vi "20211001_02.vi"() -> ()   [LabVIEW 2019]
uses:
  <vilib>/Utility/miscctls.llb/LVBoundsTypeDef.ctl
panel:
  in  "Button Size":T1={"Width"=192, "Height"=192}
  in  "Visible":bool=TRUE
  in  "Colors [4]":cluster{"Color Box":u32, "Color Box 2":u32}[](array[cluster])=[{"Color Box"=16777216, "Color Box 2"=16777216}, {"Color Box"=4424887, "Color Box 2"=4424887}, {"Color Box"=16777216, "Color Box 2"=16777216}, {"Color Box"=4424887, "Color Box 2"=4424887}]
  in  "Boolean":bool
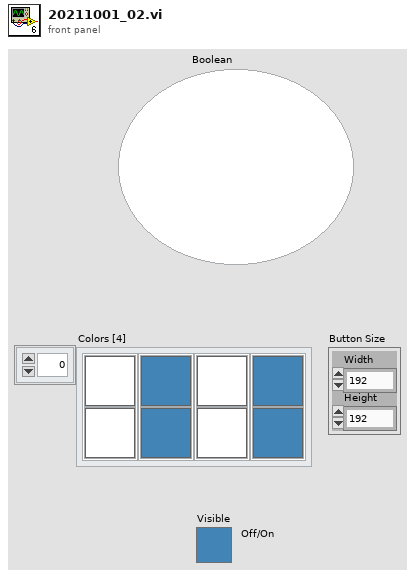
[diagram p1: front panel]
types:
  T1 = typedef "LVBoundsTypeDef.ctl" = cluster{"Width":u32, "Height":u32}
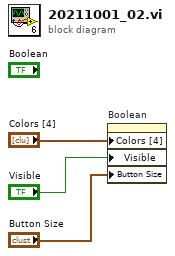
[diagram p0: block diagram]
diagram:
  n1 = property on="Boolean" class="Bool (strict)"("Colors [4]"="Colors [4]", "Visible"="Visible", "Button Size"="Button Size") -> ()  [unwired: 2 in, 2 out]
